vi "PH_PP_CurrentMeas.ProcCases.vi"(0 "i ref in":refnum<vi>, 1 "selector":string, 2 "data":T1, 3 "call cluster":T2={"Object"="", "Selector"="", "CallType"=enum."synchronous", "Async Object"="", "Async Selector"="", "Data Descriptor"="", "Data"=[], "Error #"=0, "Expire"=0}, 5 "error in":errorcluster) -> (14 "i ref out":refnum<vi>, 17 "answer cluster":T2={"Object"="", "Selector"="", "CallType"=enum."synchronous", "Async Object"="", "Async Selector"="", "Data Descriptor"="", "Data"=[], "Error #"=0, "Expire"=0}, 19 "error out":errorcluster)   [LabVIEW 2014, in "PH_PP_CurrentMeas.lvlib"]
doc: "This method is called by a process from within the default case in the event loop. The methods of a class that are linked to events will be called from THIS method. Add your code here."
uses:
  PH_PP_CurrentMeas.lvlib
  CS_Core/CSSystem/CoreDefs/CoreDefs.call_type.ctl
  CS_Core/BaseProcess/BaseProcess.descriptor string definition.ctl
  CS_Core/CSSystem/CoreDefs/CoreDefs.rawDataType.ctl
  CS_Core/CSSystem/CoreLib/CoreLib.string 2 byte array.vi
  CS_Core/BaseProcess/BaseProcess.lvlib
  CS_Core/CSSystem/CoreLib/CoreLib.lvlib
  CS_Core/CAEObj/CAEObj.lvlib
  PH_Basics/PH_PSDBWriter/PH_PSDBWriter.lvlib
  PH_Basics/PH_StatusHandler/PH_StatusHandler.lvlib
  PH_Basics/PH_Common/PH_Common.lvlib
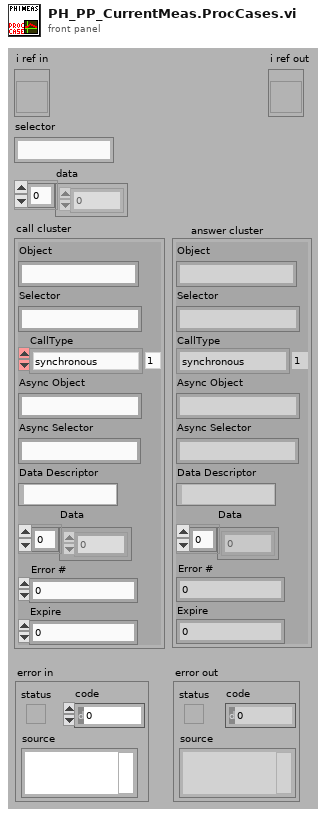
[diagram p1: front panel]
types:
  T1 = typedef "CoreDefs.rawDataType.ctl" = i8[]
  T2 = typedef "CoreDefs.call_type.ctl" = cluster{"Object":string, "Selector":string, "CallType":enum16{"simple", "synchronous", "asynchronous"}, "Async Object":string, "Async Selector":string, "Data Descriptor":T3, "Data":T1, "Error #":i32, "Expire":u32}
  T3 = typedef "BaseProcess.lvlib/BaseProcess.descriptor string definition.ctl" = string
  T4 = typedef "PH_PSDBWriter.lvlib/PH_PSDBWriter.PHELIX-Subsystems.ctl" = i32
  T5 = typedef "PH_StatusHandler.lvlib/PH_StatusHandler.Status.ctl" = i16
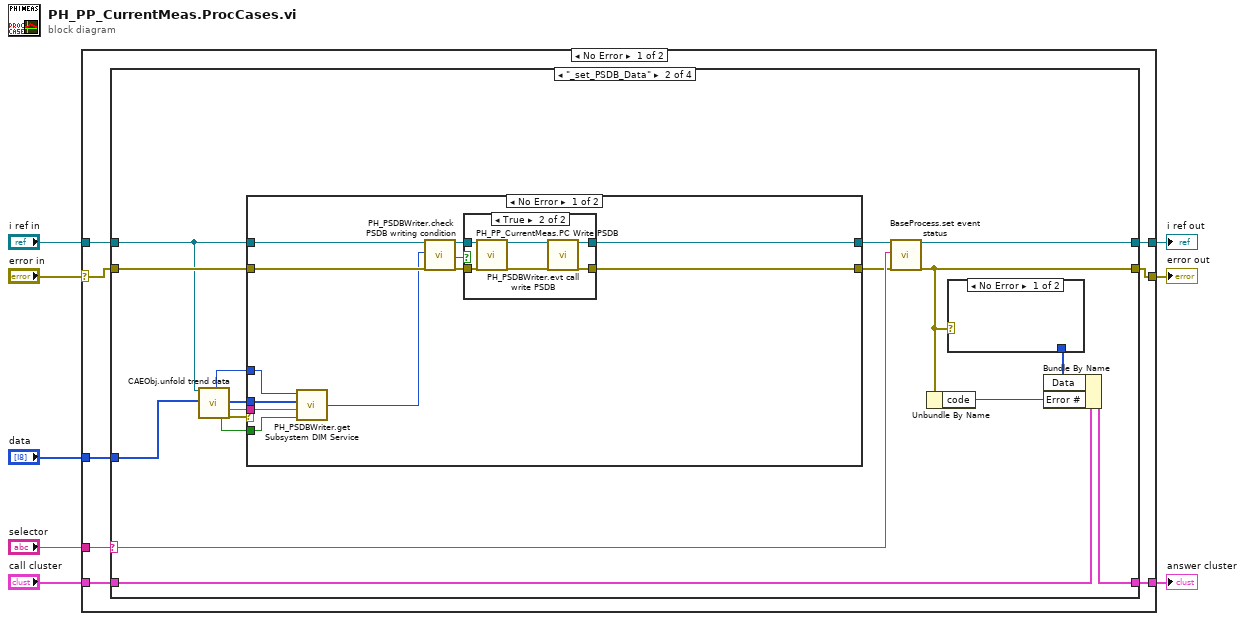
[diagram p0: block diagram]
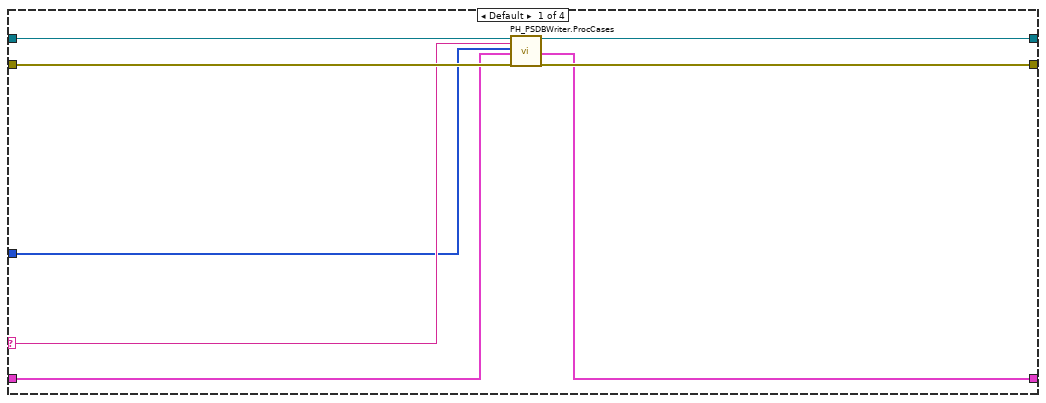
[diagram p2: hidden frame]
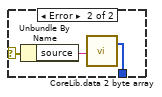
[diagram p5: hidden frame]
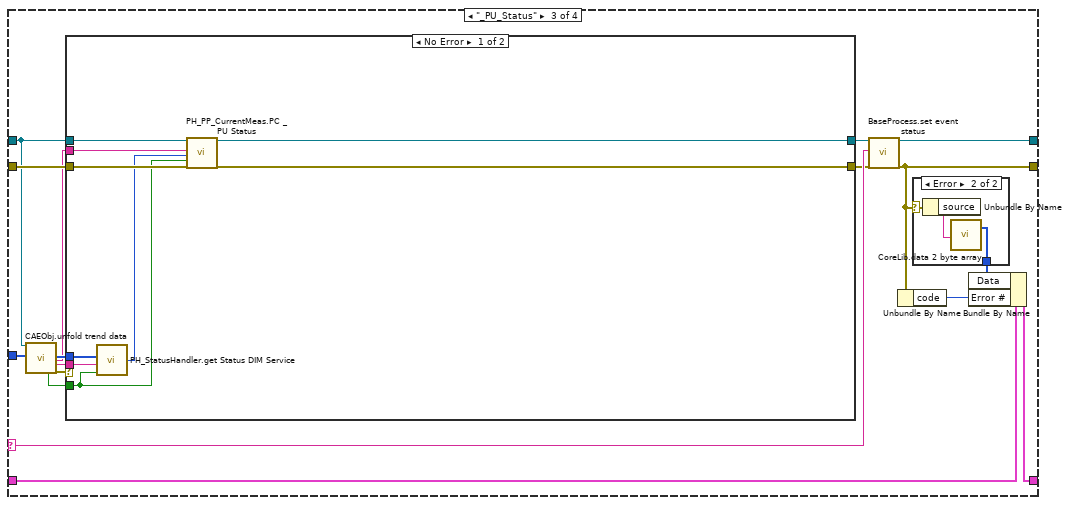
[diagram p6: hidden frame]
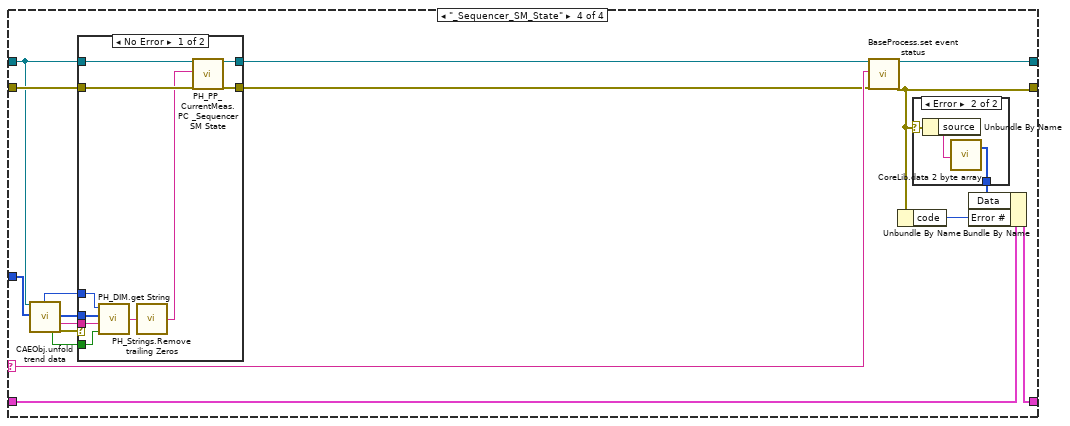
[diagram p9: hidden frame]
diagram:
  n1 = case shown="No Error" "error in" {
    selector: "error in" -> [w9 w131]
    tunnel: "selector" -> [w16 _]
    tunnel: [w15 w130] -> w7
    tunnel: "call cluster" -> [w14 w130]
    tunnel: "i ref in" -> [w13 w132]
    tunnel: [w12 w132] -> w4
    tunnel: [w10 w131] -> w3
    tunnel: "data" -> [w11 _]
    frame No Error {
      n2 = case shown="\"_set_PSDB_Data\"" w16 {
        selector: w16 -> [w19 w38 w80 w111]
        tunnel: w13 -> [w18 w27 w70 w101]
        tunnel: [w24 w37 w79 w110] -> w12
        tunnel: w14 -> [w20 w36 w78 w109]
        tunnel: [w21 w40 w82 w113] -> w15
        tunnel: w9 -> [w23 w28 w71 w102]
        tunnel: [w22 w39 w81 w112] -> w10
        tunnel: w11 -> [w17 w25 w68 w99]
        frame Default {
          n3 = call "PH_PSDBWriter.ProcCases.vi"("i ref in"=w18, "selector"=w19, "Data"=w17, "call cluster"=w20, "error in"=w23) -> ("i ref out"=w24:refnum<vi>, "answer cluster"=w21:T2, "error out"=w22:errorcluster)  [unwired: 12 in]
        }
        frame "_set_PSDB_Data" {
          n4 = call "CAEObj.unfold trend data.vi"("i ref in"=w27, "raw trend data"=w25) -> ("quality"=w30:i32, "no link"=w33:bool, "data"=w31:i8[], "typeDescriptor"=w32:string, "error out"=w34:errorcluster)  [unwired: 9 in, 4 out]
          n5 = case shown="No Error" w34 {
            tunnel: w28 -> [w53 w63]
            tunnel: [w52 w62] -> w26
            tunnel: [w51 w63] -> w29
            tunnel: w27 -> [w49 w62]
            tunnel: w33 -> [w43 _]
            tunnel: w32 -> [w45 _]
            tunnel: w31 -> [w46 _]
            tunnel: w30 -> [w44 _]
            frame No Error {
              n6 = call "PH_PSDBWriter.get Subsystem DIM Service.vi"("no link"=w43, "typeDescriptor"=w45, "data"=w46, "quality"=w44) -> ("PHELIX Subsystems"=w42:T4)
              n7 = call "PH_PSDBWriter.check PSDB writing condition.vi"("i ref in"=w49, "wanted Subsystem"=w42, "error IO"=w53) -> ("i ref out"=w48:refnum<vi>, "write PSDB?"=w47:bool, "error out"=w50:errorcluster)  [unwired: 14 in]
              n8 = case shown="True" w47 {
                tunnel: w50 -> [w54 w61]
                tunnel: [w55 w56] -> w52
                tunnel: [w54 w58] -> w51
                tunnel: w48 -> [w55 w60]
                frame False {
                }
                frame True {
                  n9 = call "PH_PP_CurrentMeas.PC Write PSDB.vi"("i ref in"=w60, "error IO"=w61) -> ("i ref out"=w57:refnum<vi>, "error out"=w59:errorcluster)  [unwired: 16 in]
                  n10 = call "PH_PSDBWriter.evt call write PSDB.vi"("i ref in"=w57, "error in (no error)"=w59) -> ("i ref out"=w56:refnum<vi>, "error out"=w58:errorcluster)  [unwired: 16 in]
                }
              }
            }
            frame Error {
            }
          }
          n11 = call "BaseProcess.set event status.vi"("i ref in"=w26, "EventStatus"=w38, "error in (no error)"=w29) -> ("i ref out"=w37:refnum<vi>, "error out"=w39:errorcluster)  [unwired: 14 in, 1 out]
          n12 = Unbundle By Name(w39) -> ("code"=w41:i32)
          n13 = case shown="No Error" w39 {
            selector: w39 -> [_ w66]
            tunnel: [_ w64] -> w35
            frame No Error {
            }
            frame Error {
              n14 = Unbundle By Name(w66) -> ("source"=w65:string)
              n15 = call-poly "CoreLib.data 2 byte array.vi"("string"=w65) -> ("byteArray out"=w64:T1)  [unwired: 18 in]
            }
          }
          n16 = Bundle By Name(cluster=w36, "Data"=w35, "Error #"=w41) -> (w40:T2)
        }
        frame "_PU_Status" {
          n17 = call "CAEObj.unfold trend data.vi"("i ref in"=w70, "raw trend data"=w68) -> ("no link"=w75:bool, "data"=w73:i8[], "serviceName"=w67:string, "typeDescriptor"=w74:string, "error out"=w76:errorcluster)  [unwired: 9 in, 4 out]
          n18 = case shown="No Error" w76 {
            tunnel: w71 -> [w88 w94]
            tunnel: [w84 w93] -> w69
            tunnel: [w85 w94] -> w72
            tunnel: w70 -> [w89 w93]
            tunnel: w75 -> [w86 _]
            tunnel: w74 -> [w91 _]
            tunnel: w73 -> [w92 _]
            tunnel: w67 -> [w90 _]
            frame No Error {
              n19 = call "PH_StatusHandler.get Status DIM Service.vi"("no link"=w86, "typeDescriptor"=w91, "data"=w92) -> ("Status"=w87:T5)  [unwired: 1 in]
              n20 = call "PH_PP_CurrentMeas.PC _PU Status.vi"("i ref in"=w89, "serviceName"=w90, "Status"=w87, "no link"=w86, "error in (no error)"=w88) -> ("i ref out"=w84:refnum<vi>, "error out"=w85:errorcluster)  [unwired: 13 in]
            }
            frame Error {
            }
          }
          n21 = call "BaseProcess.set event status.vi"("i ref in"=w69, "EventStatus"=w80, "error in (no error)"=w72) -> ("i ref out"=w79:refnum<vi>, "error out"=w81:errorcluster)  [unwired: 14 in, 1 out]
          n22 = Unbundle By Name(w81) -> ("code"=w83:i32)
          n23 = case shown="Error" w81 {
            selector: w81 -> [_ w97]
            tunnel: [_ w95] -> w77
            frame No Error {
            }
            frame Error {
              n24 = Unbundle By Name(w97) -> ("source"=w96:string)
              n25 = call-poly "CoreLib.data 2 byte array.vi"("string"=w96) -> ("byteArray out"=w95:T1)  [unwired: 18 in]
            }
          }
          n26 = Bundle By Name(cluster=w78, "Data"=w77, "Error #"=w83) -> (w82:T2)
        }
        frame "_Sequencer_SM_State" {
          n27 = call "CAEObj.unfold trend data.vi"("i ref in"=w101, "raw trend data"=w99) -> ("quality"=w98:i32, "no link"=w106:bool, "data"=w104:i8[], "typeDescriptor"=w105:string, "error out"=w107:errorcluster)  [unwired: 9 in, 4 out]
          n28 = case shown="No Error" w107 {
            tunnel: w102 -> [w123 w126]
            tunnel: [w117 w125] -> w100
            tunnel: [w118 w126] -> w103
            tunnel: w101 -> [w124 w125]
            tunnel: w106 -> [w122 _]
            tunnel: w105 -> [w121 _]
            tunnel: w104 -> [w120 _]
            tunnel: w98 -> [w115 _]
            frame No Error {
              n29 = call "PH_DIM.get String.vi"("no link"=w122, "typeDescriptor"=w121, "data"=w120, "quality"=w115) -> ("Output String"=w119:string)
              n30 = call "PH_Strings.Remove trailing Zeros.vi"("Input String"=w119) -> ("Output String"=w116:string)
              n31 = call "PH_PP_CurrentMeas.PC _Sequencer SM State.vi"("i ref in"=w124, "Sequencer SM State"=w116, "error in (no error)"=w123) -> ("i ref out"=w117:refnum<vi>, "error out"=w118:errorcluster)  [unwired: 15 in]
            }
            frame Error {
            }
          }
          n32 = call "BaseProcess.set event status.vi"("i ref in"=w100, "EventStatus"=w111, "error in (no error)"=w103) -> ("i ref out"=w110:refnum<vi>, "error out"=w112:errorcluster)  [unwired: 14 in, 1 out]
          n33 = Unbundle By Name(w112) -> ("code"=w114:i32)
          n34 = case shown="Error" w112 {
            selector: w112 -> [_ w129]
            tunnel: [_ w127] -> w108
            frame No Error {
            }
            frame Error {
              n35 = Unbundle By Name(w129) -> ("source"=w128:string)
              n36 = call-poly "CoreLib.data 2 byte array.vi"("string"=w128) -> ("byteArray out"=w127:T1)  [unwired: 18 in]
            }
          }
          n37 = Bundle By Name(cluster=w109, "Data"=w108, "Error #"=w114) -> (w113:T2)
        }
      }
    }
    frame Error {
    }
  }
  "answer cluster" <- w7
  "i ref out" <- w4
  "error out" <- w3
